vi "RelayOpen_R.vi"(0 "datain":string[](array[string])=["备注", "负载通道", "负载地址", "延时时间", "output max", "output min", "量测类型", "待测物板号"], 5 "HW CH Number":i32=4, 7 "Setup":string) -> (4 "REPORT INDECATE":string[][](array[string])=[["微安测试", "", "", "", ""], ["微安量测", "4", "0.000", "0.1", "NG"], ["微安量测", "4", "0.000", "0.1", "NG"], ["微安量测", "4", "0.000", "0.1", "NG"], ["微安量测", "4", "0.000", "0.1", "NG"]], 6 "ROW HEAD":string[](array[string]), 8 "PF":string[](array[string]), 10 "testData":string[](array[string]), 14 "数组":bool[](array[boolean]), 15 "Array":string[](array[string]))   [LabVIEW 2018]
uses:
  Subvi/Global.vi
panel:
  out "OpenStr2":string
  out "cmd":string[](array[string])
  out "测试板数":i32=4
  # "[VoltageTest]\nExt.Name =2222222222;\nAddress =1;\nDelay Time =1;\nMAX.Spec =*;\nMin.Spec =2;\nTest Type =;\nRelayH_8Bit =0,0,0,0;\nRelayL_8Bit =0,0,0,0;\nStart board number =1;#"
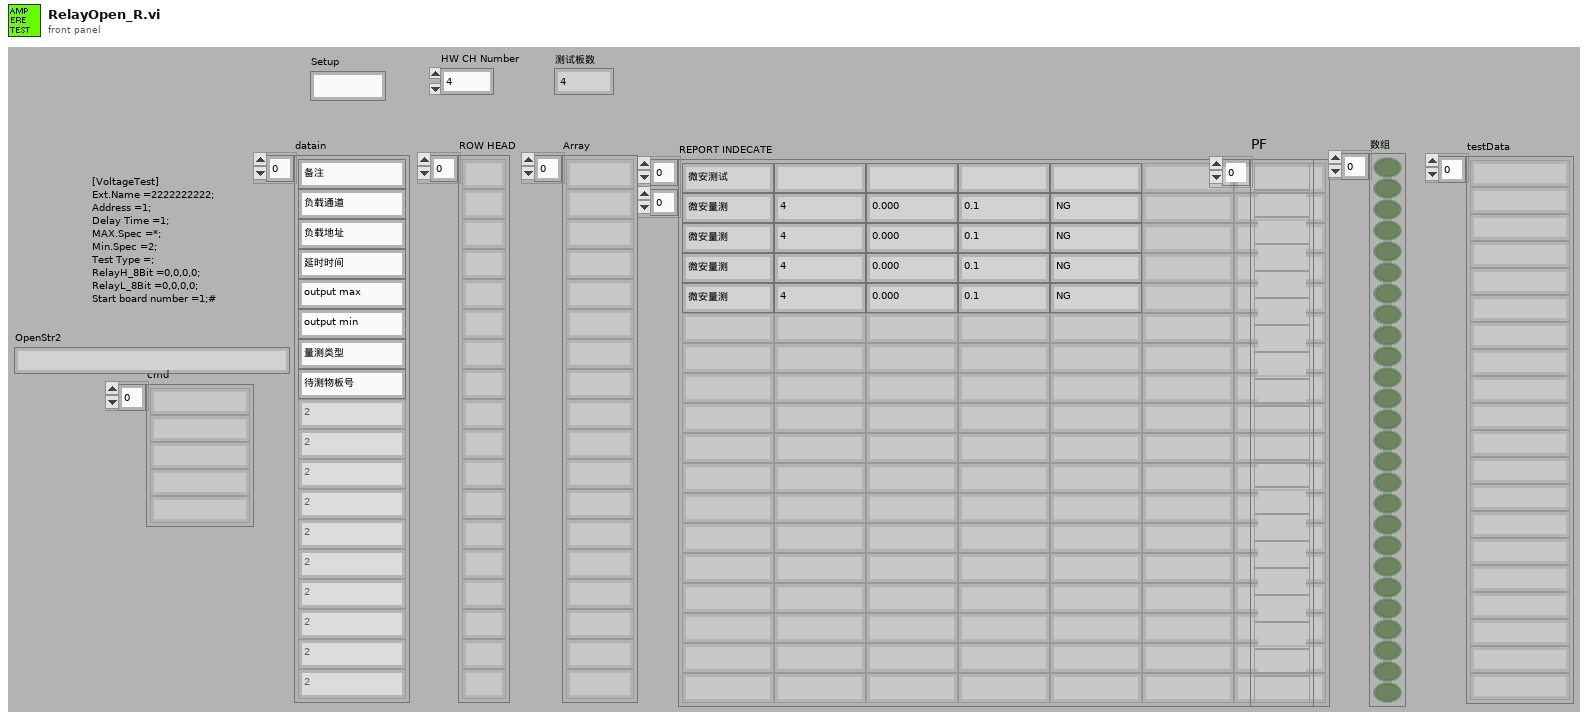
[diagram p1: front panel]
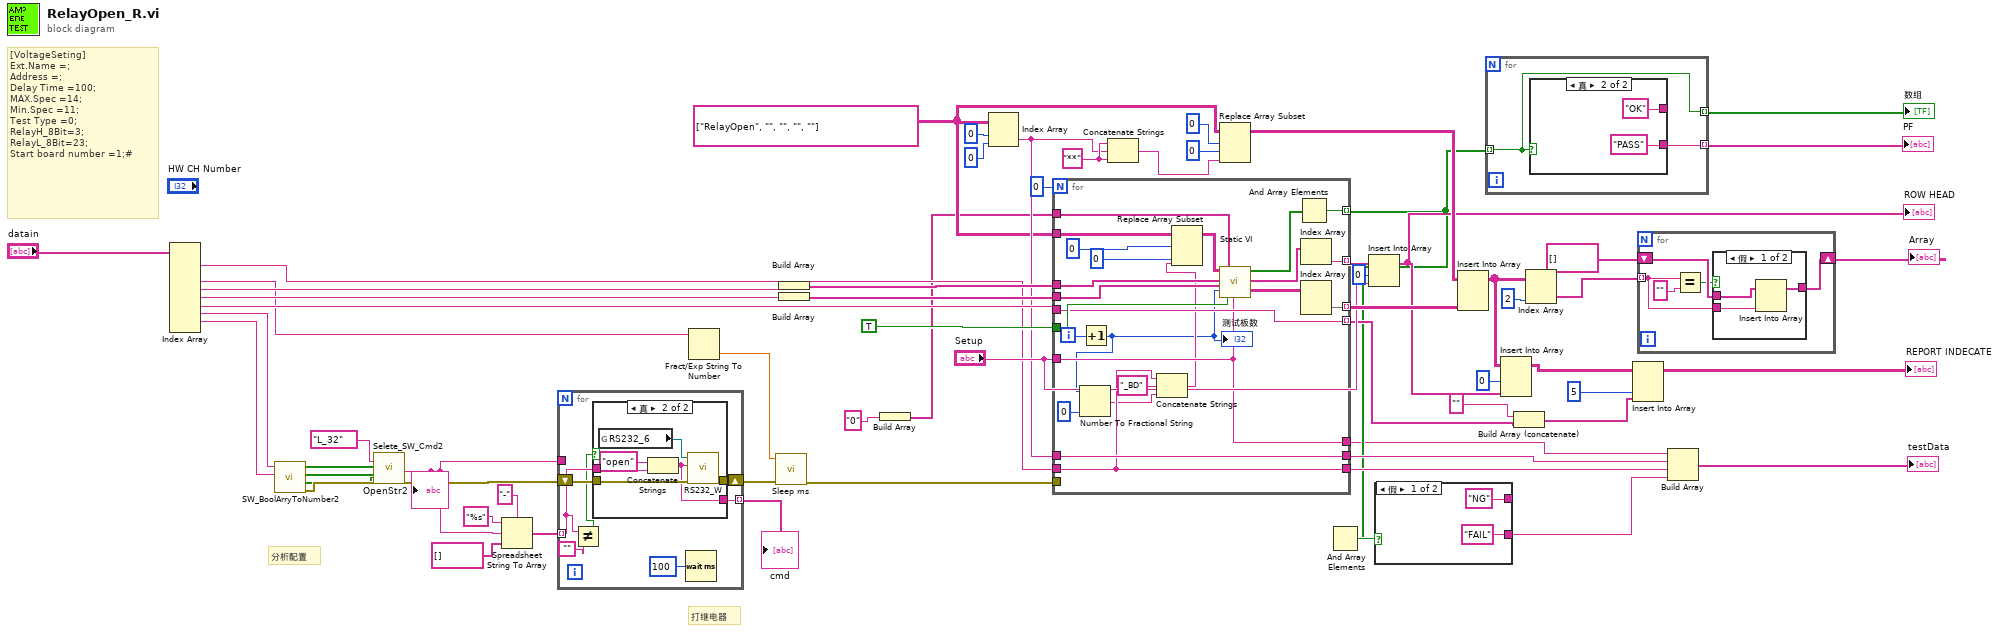
[diagram p0: block diagram]
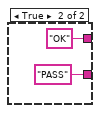
[diagram p3: hidden frame]
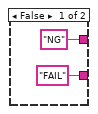
[diagram p4: hidden frame]
diagram:
  w22 = string[][] [["RelayOpen", "", "", "", ""]]
  w56 = "**" ("字符串")
  # "分析配置"
  # "打继电器"
  # "[VoltageSeting]\nExt.Name =;\nAddress =;\nDelay Time =100;\nMAX.Spec =14;\nMin.Spec =11;\nTest Type =0;\nRelayH_8Bit=3;\nRelayL_8Bit=23;\nStart board number =1;#"
  n1 = Index Array(array="datain") -> (element #1=w23:string, element #3=w16:string, element #4=w52:string, element #5=w51:string, element #6=w39:string, element #7=w15:string, element #8=w14:string)  [unwired: 9 in, 2 out]
  n2 = call "SW_BoolArryToNumber2.vi"("L32 INUPT"=w14, "H32 INUPT"=w15) -> ("error out"=w10:errorcluster, "64 SW OUT"=w7:bool[], "L_32"=w12:bool[], "H_32"=w18:bool[])  [unwired: 6 in]
  n3 = call "Selete_SW_Cmd2.vi"("组合框"="L_32", "H_32"=w18, "L_32"=w12, "64 SW OUT"=w7, "error in (no error)"=w10) -> ("OpenStr2"=w1:string, "error out"=w9:errorcluster)  [unwired: 11 in, 2 out]
  "OpenStr2" <- w1
  n4 = Spreadsheet String To Array(delimiter (Tab)="-" ("分隔符(Tab)"), format string="%s" ("格式字符串"), spreadsheet string=w1, array type (2D Dbl)=string[] []) -> (array=w3:string[])
  n5 = for {
    tunnel: w1 -> [_]
    shift-right: [w70] -> w8
    shift-left: w9 -> [w71]
    tunnel: w3 -> [w68] mode=indexing
    tunnel: [w65] -> w2 mode=indexing
    n6 = Not Equal?(x=w68, y="") -> (x != y?=w66:bool)
    n7 = case shown="真" w66 {
      tunnel: w71 -> [w72 w78]
      tunnel: [w72 w77] -> w70
      tunnel: w68 -> [_ w74]
      tunnel: [_ w73] -> w65
      frame False {
      }
      frame True {
        n8 = global read "Global.vi" "RS232_6"() -> (w76:refnum<visa-resource-name>)
        n9 = Concatenate Strings("open", w74) -> (w73:string)
        n10 = call "RS232_W.vi"("error in (no error)"=w78, "CMD"=w73, "VISA资源名称"=w76) -> ("error out"=w77:errorcluster)  [unwired: 6 in, 2 out]
      }
    }
    n11 = Wait (ms)(milliseconds to wait=u32 100 ("等待时间（毫秒）")) -> ()  [unwired: 1 out]
  }
  "cmd" <- w2
  n12 = Fract/Exp String To Number(string=w16) -> (number=w17:dbl)  [unwired: 3 in, 1 out]
  n13 = call "Sleep ms.vi"("error in (no error)"=w8, "等待时间（毫秒）"=w17) -> ("error out"=w13:errorcluster)  [unwired: 9 in]
  n14 = Build Array(w52) -> (w50:string[])
  n15 = Build Array(w51) -> (w49:string[])
  n16 = Build Array("0") -> (w19:string[])
  n17 = Index Array(array=w22, index (row)=0 ("索引 (行)"), index (col)=0 ("禁用的索引 (列)")) -> (element=w32:string)
  n18 = for {
    N: 0 -> [_]
    tunnel: w19 -> [w102]
    tunnel: w50 -> [w101]
    tunnel: w49 -> [w100]
    tunnel: "Setup" -> [w90]
    tunnel: TRUE -> [w98]
    tunnel: [w97] -> w28 mode=indexing
    tunnel: [w95] -> w45 mode=indexing
    tunnel: [w93] -> w46 mode=indexing
    tunnel: w39 -> [w92]
    tunnel: [w92] -> w35 mode=indexing
    tunnel: w32 -> [w91]
    tunnel: [w91] -> w31
    tunnel: w23 -> [w82]
    tunnel: [w82] -> w30
    tunnel: [w90] -> w25
    tunnel: w22 -> [w88]
    tunnel: w13 -> [_]
    i -> [w85]
    n19 = Increment(x=w85) -> (x+1=w79:i32)
    "测试板数" <- w79
    n20 = Number To Fractional String(number=w79, precision (6)=i16 0 ("精度(6)")) -> (F-format string=w81:string)  [unwired: 2 in]
    n21 = Concatenate Strings(w82, "_BD" ("字符串"), w81) -> (w80:string)
    n22 = Replace Array Subset(array=w88, new element=w80, index (row)=0 ("索引 (行)"), index (col)=0 ("禁用的索引 (列)")) -> (w87:string[][])
    n23 = call "Static VI.vi"("添加的数组"=w87, "Max"=w101, "Min"=w100, "板数"=w79, "INPUTSTRING"=w102, "是否为字符串对比"=w98, "SQ"=w90) -> ("P/F"=w99:bool[], "SQ out"=w96:string[], "arrauy out"=w94:string[][])  [unwired: 9 in, 1 out]
    n24 = And Array Elements(Boolean array=w99) -> (logical AND=w97:bool)
    n25 = Index Array(array=w96) -> (element=w95:string)  [unwired: 1 in]
    n26 = Index Array(array=w94) -> (element=w93:string[])  [unwired: 2 in]
  }
  n27 = Concatenate Strings(w56, w32, w56) -> (w53:string)
  n28 = Replace Array Subset(array=w22, new element=w53, index (row)=0 ("索引 (行)"), index (col)=0 ("禁用的索引 (列)")) -> (w47:string[][])
  n29 = And Array Elements(Boolean array=w28) -> (logical AND=w29:bool)
  n30 = Insert Into Array(array=w45, index=0 ("索引"), new element="Setup") -> (w41:string[])
  "ROW HEAD" <- w41
  n31 = case shown="假" w29 {
    tunnel: ["NG" "OK"] -> _
    tunnel: ["FAIL" "PASS"] -> w27
    frame False {
    }
    frame True {
    }
  }
  n32 = Insert Into Array ("数组插入")(array=w47, new element=w46) -> (w42:string[][])  [unwired: 2 in]
  n33 = for {
    tunnel: w28 -> [w107] mode=indexing
    tunnel: [w108] -> w60 mode=indexing
    tunnel: [w107] -> w24 mode=indexing
    n34 = case shown="真" w107 {
      tunnel: ["NG" "OK"] -> _
      tunnel: ["FAIL" "PASS"] -> w108
      frame False {
      }
      frame True {
      }
    }
  }
  "PF" <- w60
  "数组" <- w24
  n35 = Insert Into Array(array=w42, index (col)=0 ("禁用的索引 (列)"), new element=w41) -> (w37:string[][])  [unwired: 1 in]
  n36 = Build Array (concatenate)("" ("字符串"), w35) -> (w33:string[])
  n37 = Index Array(array=w42, index (col)=2 ("禁用的索引 (列)")) -> (element=w62:string[])  [unwired: 1 in]
  n38 = Insert Into Array(array=w37, index (col)=5 ("禁用的索引 (列)"), new element=w33) -> (→"REPORT INDECATE":string[][])  [unwired: 1 in]
  n39 = for {
    tunnel: w62 -> [w113] mode=indexing
    shift-right: [w114] -> w61
    shift-left: string[] [] ("Array") -> [w117]
    n40 = Equal?(x=w113, y="") -> (x = y?=w115:bool)
    n41 = case shown="假" w115 {
      tunnel: w117 -> [w120 w121]
      tunnel: [w119 w121] -> w114
      tunnel: w113 -> [w118 _]
      frame False {
        n42 = Insert Into Array(array=w120, new element=w118) -> (w119:string[])  [unwired: 1 in]
      }
      frame True {
      }
    }
  }
  "Array" <- w61
  n43 = Build Array(w25, w31, w30, w27) -> (→"testData":string[])
